vi "force sensor1.vi"   [LabVIEW 2010, in "Rampage.lvrbt"]
uses:
  Rampage.lvrbt
  <vilib>/NXT/Subs/MotorOutput.ctl
  <vilib>/NXT/Block Support/NXT_InputPort.ctl
  <vilib>/NXT/Dual Mode Library/Motors/oldLightOn.vi
types:
  T1 = typedef "MotorOutput.ctl" = u8
  T2 = typedef "NXT_InputPort.ctl" = u8
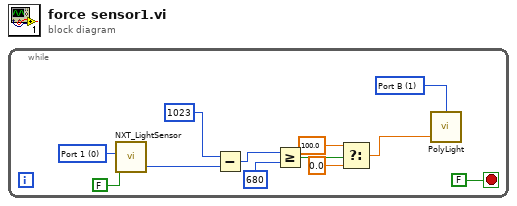
[diagram p0: block diagram]
diagram:
  n1 = while {
    stop <- FALSE stop-if-true
    w1 = T1 1 items=["Port A"=0, "Port B"=1, "Port C"=2, "Ports A & B"=4, "Ports A & C"=5, "Ports B & C"=6, "All Ports"=3] ("Output Port (All Ports)")
    w12 = T2 0 items=["Port 1", "Port 2", "Port 3", "Port 4"] ("Input (Port 3)")
    n2 = call <vilib>:"NXT_LightSensor.vi"("Floodlight"=FALSE, "Input (Port 3)"=w12) -> ("Raw Value"=w11:u16)  [unwired: 6 in, 3 out]
    n3 = Subtract(x=u16 1023, y=w11) -> (x-y=w7:u16)
    n4 = Greater Or Equal?(x=w7, y=u16 680) -> (x >= y?=w5:bool)
    n5 = Select(t=100.0, s=w5, f=0.0) -> (s? t:f=w2:dbl)
    n6 = call-poly <vilib>:"PolyLight.vi"("Power (75)"=w2, "Output Port (All Ports)"=w1) -> ()  [unwired: 2 in, 1 out]
  }
